vi "Teleop v1a.vi"(10 "Match Info":T1={"Autonomous Elapsed Seconds"=0.0, "TeleOp Elapsed Seconds"=0.0, "Disabled Elapsed Seconds"=0.0, "Visited Autonomous"=FALSE, "Visited TeleOp"=FALSE, "Visited Disabled"=FALSE, "Autonomous Settings"={"Autonomous Style"=enum."Independent", "VI Refnum"=refnum}}, 11 "Call Context":T2) -> ()   [LabVIEW 2019]
doc: "This VI is called for each TeleOp packet received from the DS where the robot is not disabled. It is often used to read from the joysticks and update I/O or to update setpoints for timed control loops. It should complete and return within 20 milliseconds or it may miss DS packets."
uses:
  <vilib>/Rock Robotics/WPI/DriverStation/WPI_DriverStationDerivedRobotMode.ctl
  <vilib>/Rock Robotics/WPI/DriverStation/WPI_DriverStationMatch Info.ctl
  <vilib>/Rock Robotics/WPI/Relay/WPI_RelayValue.ctl
  <vilib>/Rock Robotics/WPI/Utilities/WPI_GetSetVariantRefNum.vi
  <vilib>/Rock Robotics/Network Tables/NT Write Boolean Array.vi
  <vilib>/Rock Robotics/Network Tables/NT Write Numeric Array.vi
  <vilib>/Rock Robotics/Network Tables/NT Read Boolean.vi
  <vilib>/Rock Robotics/Network Tables/NT Read Number.vi
panel:
  out "Sample Slider 0":dbl(slide) scale=0.0..5.0
  out "Sample Boolean 1":bool
  out "Sample Boolean 0":bool
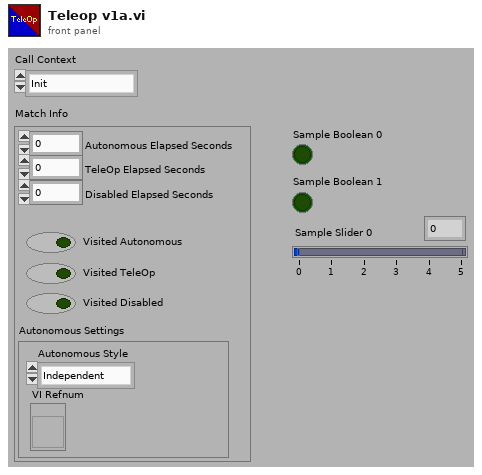
[diagram p1: front panel]
types:
  T1 = typedef "WPI_DriverStationMatch Info.ctl" = cluster{"Autonomous Elapsed Seconds":dbl, "TeleOp Elapsed Seconds":dbl, "Disabled Elapsed Seconds":dbl, "Visited Autonomous":bool, "Visited TeleOp":bool, "Visited Disabled":bool, "Autonomous Settings":cluster{"Autonomous Style":enum16{"Iterative", "Independent"}, "VI Refnum":refnum<vi>}}
  T2 = typedef "WPI_DriverStationDerivedRobotMode.ctl" = enum16{"Init", "Execute", "Stop"}
  T3 = typedef "WPI_RobotDriveDevRef.ctl" = cluster{"DevStatus":errorcluster, "Motors[]":T4[], "Square Inputs":bool, "Max Output":dbl}
  T4 = typedef "WPI_MotorControlDeviceRef.ctl" = cluster{"DeviceStatus":errorcluster, "Type":T5, "PWM":cluster{"PWM Channel":T6, "DeadBand":T7}, "CAN":cluster{"Device Number":u8, "SetOutput VI Ref":variant, "GetOutput VI Ref":variant, "Enable VI Ref":variant, "Disable VI Ref":variant, "Data":variant}, "Invert":bool, "DIO PWM":cluster{"PWM \"Enable\" Channel":T6, "DIOChannel":T8, "PWM Rate":dbl}}
  T5 = typedef "WPI_MotorControlType.ctl" = enum16{"PWM", "CAN", "DIO PWM"}
  T6 = typedef "FPGA_DIOPWMChannel.ctl" = enum8{"PWM 0", "PWM 1", "PWM 2", "PWM 3", "PWM 4", "PWM 5", "PWM 6", "PWM 7", "PWM 8", "PWM 9", "PWM MXP 0", "PWM MXP 1", "PWM MXP 2", "PWM MXP 3", "PWM MXP 4", "PWM MXP 5", "PWM MXP 6", "PWM MXP 7", "PWM MXP 8", "PWM MXP 9", "Invalid"}
  T7 = typedef "WPI_PWMDeadband.ctl" = cluster{"Name":string, "maxPositivePwm":i32, "minPositivePwm":i32, "centerPwm":i32, "maxNegativePwm":i32, "minNegativePwm":i32, "angularRange":u16}
  T8 = typedef "FPGA_DIOChannel.ctl" = enum8{"DIO 0", "DIO 1", "DIO 2", "DIO 3", "DIO 4", "DIO 5", "DIO 6", "DIO 7", "DIO 8", "DIO 9", "DIO MXP 0", "DIO MXP 1", "DIO MXP 2", "DIO MXP 3", "DIO MXP 4", "DIO MXP 5", "DIO MXP 6", "DIO MXP 7", "DIO MXP 8", "DIO MXP 9", "DIO MXP 10", "DIO MXP 11", "DIO MXP 12", "DIO MXP 13", "DIO MXP 14", "DIO MXP 15", "SPI Port CS1", "SPI Port CS2", "SPI Port CS3", "SPI Port MISO", "SPI Port MOSI", "Invalid"}
  T9 = typedef "WPI_JoystickDevRef.ctl" = cluster{"Device":T10}
  T10 = typedef "WPI_JoystickDeviceEnum.ctl" = enum16{"USB 0", "USB 1", "USB 2", "USB 3", "USB 4", "USB 5"}
  T11 = typedef "WPI_DigitalInputDevRef.ctl" = cluster{"DevStatus":errorcluster, "DIO Channel":T8}
  T12 = typedef "WPI_RelayValue.ctl" = enum16{"Off", "On", "Forward", "Reverse"}
  T13 = typedef "WPI_RelayDevRef.ctl" = cluster{"DevStatus":errorcluster, "Relay Channel":T14, "Relay Direction":T15}
  T14 = typedef "FPGA_DIORelayChannel.ctl" = enum8{"Relay 0", "Relay 1", "Relay 2", "Relay 3", "Invalid"}
  T15 = typedef "WPI_RelayDirection.ctl" = enum16{"Both directions", "Forward only", "Reverse only"}
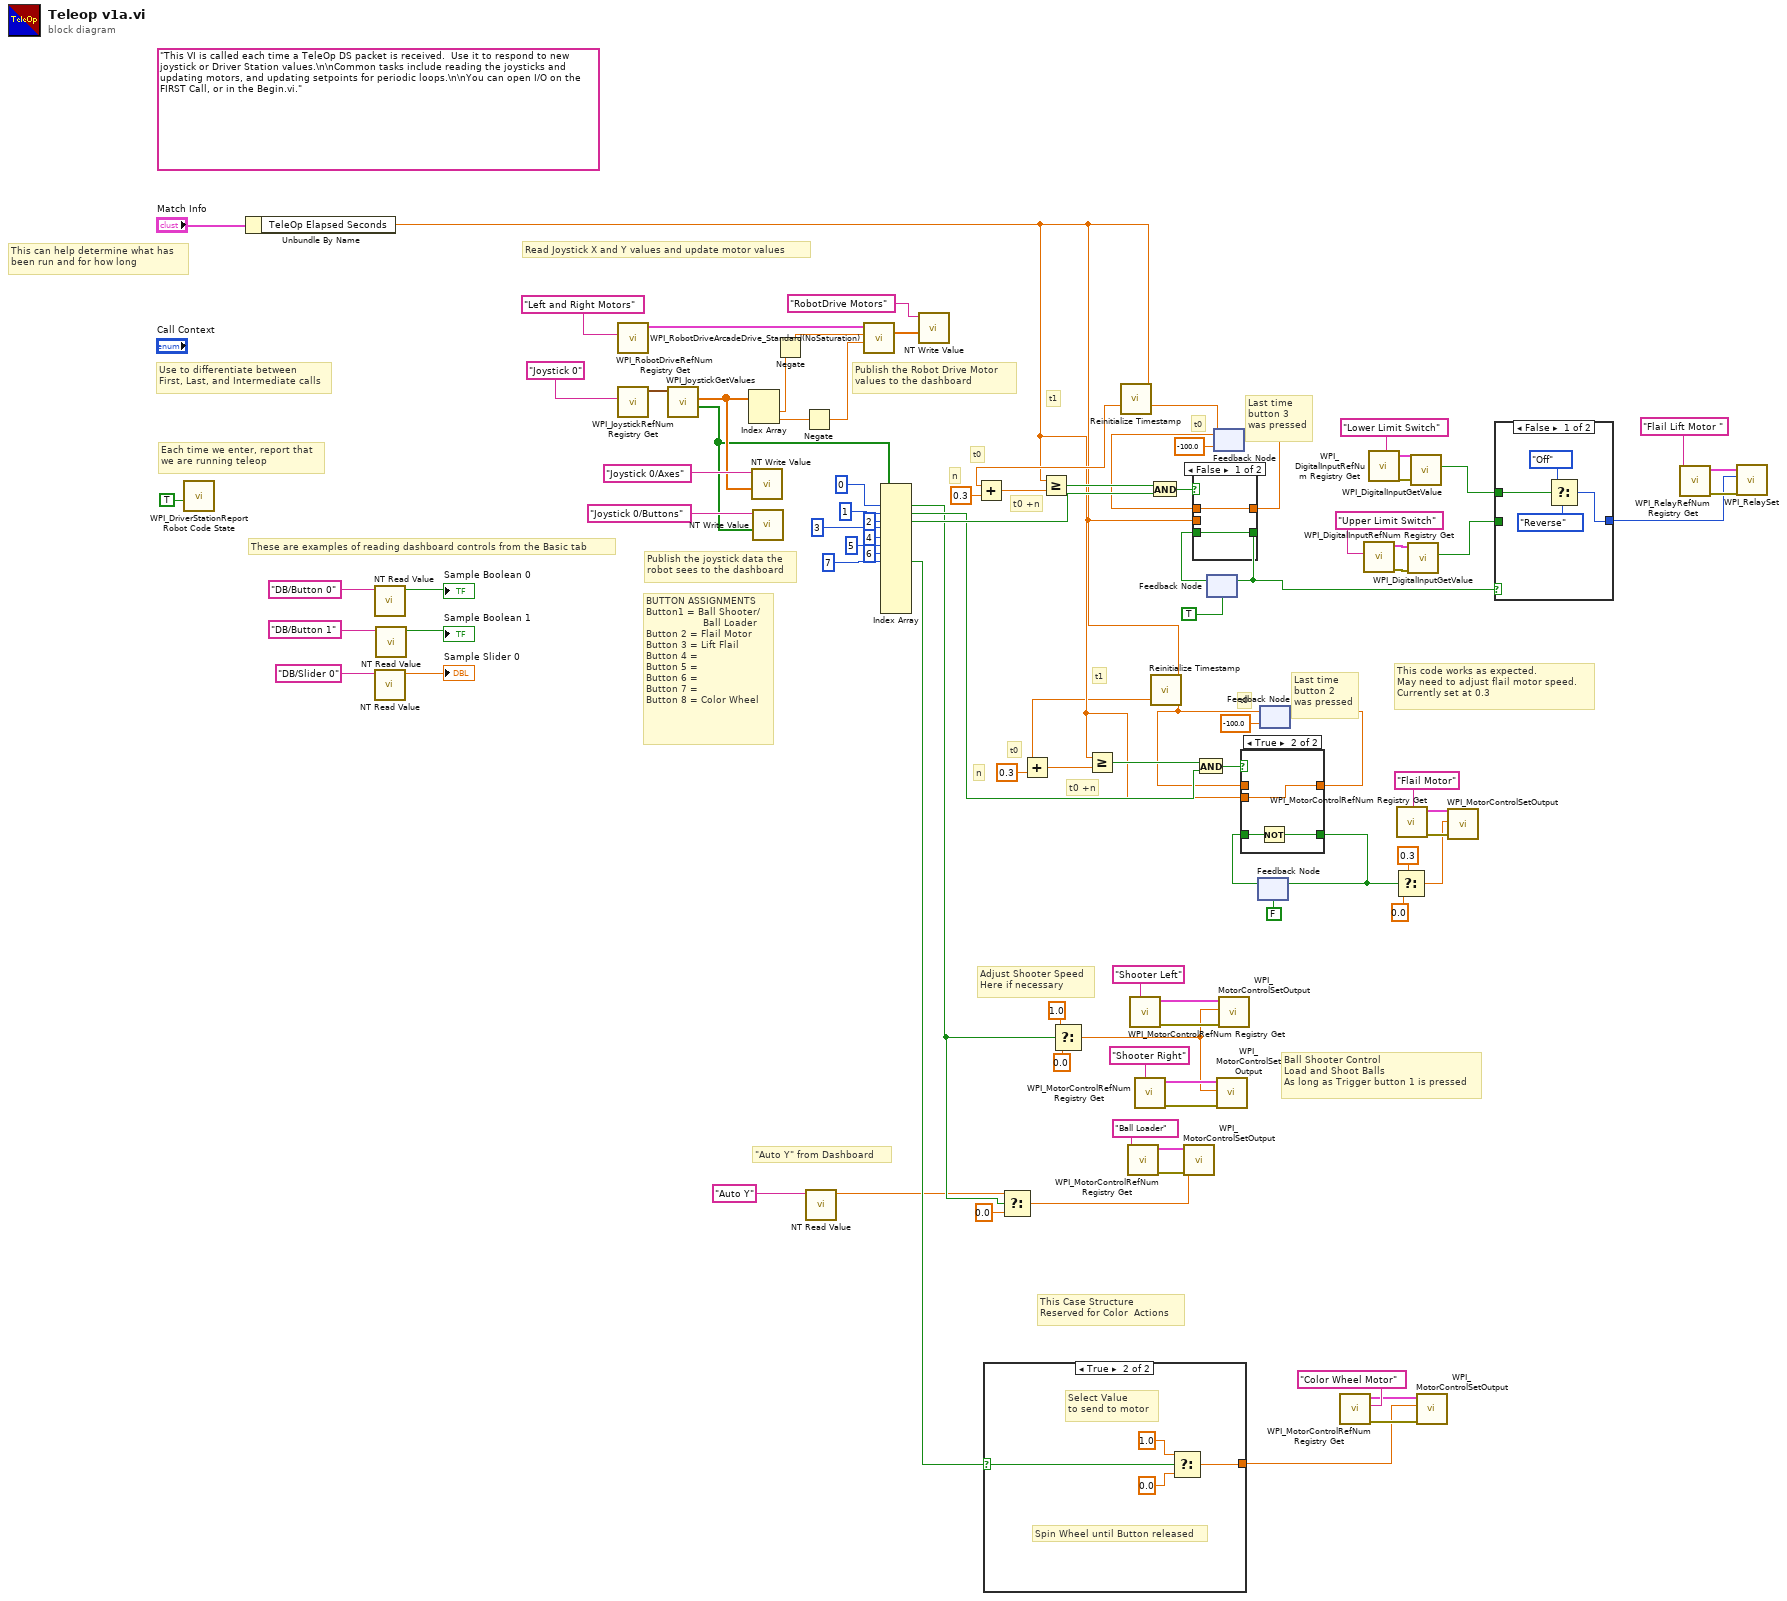
[diagram p0: block diagram]
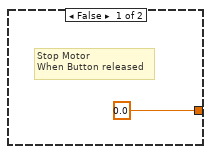
[diagram p2: hidden frame]
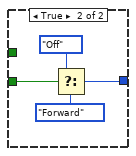
[diagram p4: hidden frame]
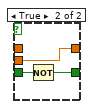
[diagram p5: hidden frame]
diagram:
  (unwired) "This VI is called each time a TeleOp DS packet is received.  Use it to respond to new joystick or Driver Station values.\n\nCommon tasks include reading the joysticks and updating motors, and updating setpoints for periodic loops.\n\nYou can open I/O on the FIRST Call, or in the Begin.vi."
  # "\"Auto Y\" from Dashboard"
  # "This Case Structure\nReserved for Color  Actions"
  # "Adjust Shooter Speed\nHere if necessary"
  # "Ball Shooter Control\nLoad and Shoot Balls \nAs long as Trigger button 1 is pressed"
  # "BUTTON ASSIGNMENTS\nButton1 = Ball Shooter/\n                   Ball Loader\nButton 2 = Flail Motor\nButton 3 = Lift Flail\nButton 4 =\nButton 5 = \nButton 6 =\nButton 7 =\nButton 8 = Color Wheel"
  # "This code works as expected.\nMay need to adjust flail motor speed.\nCurrently set at 0.3"
  # "n"
  # "t0"
  # "t0 +n"
  # "t0"
  # "t1"
  # "Last time \nbutton 2\nwas pressed"
  # "n"
  # "t0"
  # "t0 +n"
  # "t0"
  # "t1"
  # "Last time \nbutton 3\nwas pressed"
  # "These are examples of reading dashboard controls from the Basic tab"
  # "Publish the Robot Drive Motor\nvalues to the dashboard"
  # "Publish the joystick data the\nrobot sees to the dashboard"
  # "Each time we enter, report that\nwe are running teleop"
  # "Use to differentiate between\nFirst, Last, and Intermediate calls"
  # "This can help determine what has\nbeen run and for how long"
  # "Read Joystick X and Y values and update motor values"
  n1 = call <vilib>:"WPI_DriverStationReport Robot Code State.vi"("TeleOp"=TRUE ("Autonomous")) -> ()  [unwired: 10 in, 1 out]
  n2 = Unbundle By Name("Match Info") -> ("TeleOp Elapsed Seconds"=w6:dbl)
  n3 = call-poly <vilib>:"NT Read Value.vi"("Name"="DB/Button 0" ("refnum name")) -> ("Boolean"=→"Sample Boolean 0":bool)  [unwired: 9 in, 1 out]
  n4 = call-poly <vilib>:"NT Read Value.vi"("Name"="DB/Slider 0" ("refnum name")) -> ("Numeric"=→"Sample Slider 0":dbl)  [unwired: 9 in, 1 out]
  n5 = call-poly <vilib>:"NT Read Value.vi"("Name"="DB/Button 1" ("refnum name")) -> ("Boolean"=→"Sample Boolean 1":bool)  [unwired: 9 in, 1 out]
  n6 = call <vilib>:"WPI_RobotDriveRefNum Registry Get.vi"("refnum name"="Left and Right Motors") -> ("RobotDriveDevRef"=w93:T3)  [unwired: 1 in, 9 out]
  n7 = call <vilib>:"WPI_JoystickRefNum Registry Get.vi"("refnum name"="Joystick 0") -> ("JoystickDevRef"=w91:T9)  [unwired: 1 in, 9 out]
  n8 = call <vilib>:"WPI_JoystickGetValues.vi"("JoystickDevRef"=w91) -> ("Buttons"=w78:bool[], "Axes"=w87:dbl[])  [unwired: 6 in, 3 out]
  n9 = Index Array(array=w87) -> (element #1=w76:dbl, element #2=w75:dbl)  [unwired: 2 in]
  n10 = call-poly <vilib>:"NT Write Value.vi"("Numeric Array"=w87, "Name"="Joystick 0/Axes") -> ()  [unwired: 9 in, 1 out]
  n11 = call-poly <vilib>:"NT Write Value.vi"("Boolean Array"=w78, "Name"="Joystick 0/Buttons") -> ()  [unwired: 9 in, 1 out]
  n12 = Negate(x=w76) -> (-x=w2:dbl)
  n13 = Negate(x=w75) -> (-x=w3:dbl)
  n14 = call-poly <vilib>:"NT Read Value.vi"("Name"="Auto Y") -> ("Numeric"=w1:dbl)  [unwired: 9 in, 1 out]
  n15 = call <vilib>:"WPI_RobotDriveArcadeDrive_Standard(NoSaturation).vi"("Y axis value"=w3, "X axis value"=w2, "RobotDriveDevRef"=w93) -> ("Motor Values"=w80:dbl[])  [unwired: 1 in, 7 out]
  n16 = Index Array(array=w78, index #1=0 ("index"), index #2=1 ("index"), index #3=2 ("index"), index #4=3 ("index"), index #5=4 ("index"), index #6=5 ("index"), index #7=6 ("index"), index #8=7 ("index")) -> (element #1=w23:bool, element #2=w35:bool, element #3=w67:bool, element #8=w12:bool)  [unwired: 6 in, 10 out]
  n17 = call-poly <vilib>:"NT Write Value.vi"("Numeric Array"=w80, "Name"="RobotDrive Motors") -> ()  [unwired: 9 in, 1 out]
  n18 = case shown="True" w12 {
    selector: w12 -> [_ w100]
    tunnel: [0.0 ("f") w97] -> w18
    frame False {
      # "Stop Motor\nWhen Button released"
    }
    frame True {
      # "Spin Wheel until Button released"
      # "Select Value \nto send to motor"
      n19 = Select(t=1.0, s=w100, f=0.0) -> (s? t:f=w97:dbl)
    }
  }
  n20 = Select(t=w1, s=w23, f=0.0) -> (s? t:f=w9:dbl)
  n21 = Select(t=1.0, s=w23, f=0.0) -> (s? t:f=w28:dbl)
  n22 = call <vilib>:"WPI_MotorControlRefNum Registry Get.vi"("refnum name"="Ball Loader") -> ("error out"=w25:errorcluster, "MotorControlDevRef"=w24:T4)  [unwired: 9 in]
  n23 = call <vilib>:"WPI_MotorControlRefNum Registry Get.vi"("refnum name"="Shooter Left") -> ("error out"=w34:errorcluster, "MotorControlDevRef"=w33:T4)  [unwired: 9 in]
  n24 = call <vilib>:"WPI_MotorControlRefNum Registry Get.vi"("refnum name"="Shooter Right") -> ("error out"=w31:errorcluster, "MotorControlDevRef"=w30:T4)  [unwired: 9 in]
  n25 = call <vilib>:"WPI_MotorControlSetOutput.vi"("error in (no error)"=w25, "Output"=w9, "MotorControlDevRef"=w24) -> ()  [unwired: 6 in, 3 out]
  n26 = feedback #1(TRUE) -> (w73:bool)
  n27 = feedback #2(-100.0 ("TeleOp Elapsed Seconds")) -> (w7:dbl)
  n28 = call "Reinitialize Timestamp.vi"("t0 Input"=w7, "t1 Input"=w6) -> ("t0 Output"=w8:dbl)  [unwired: 9 in]
  n29 = Add(x=w8, y=0.3) -> (x+y=w65:dbl)
  n30 = Greater Or Equal?(x=w6, y=w65) -> (x >= y?=w62:bool)
  n31 = And(x=w62, y=w67) -> (x .and. y?=w66:bool)
  n32 = case shown="False" w66 {
    tunnel: [w102 w105] -> w52
    tunnel: w73 -> [w102 w104]
    tunnel: w7 -> [w101 _]
    tunnel: [w101 w103] -> w68
    tunnel: w6 -> [_ w103]
    frame False {
    }
    frame True {
      n33 = Not(x=w104) -> (.not. x?=w105:bool)
    }
  }
  n34 = feedback-in #1(w52) -> ()
  n35 = feedback-in #2(w68) -> ()
  n36 = call <vilib>:"WPI_MotorControlSetOutput.vi"("error in (no error)"=w31, "Output"=w28, "MotorControlDevRef"=w30) -> ()  [unwired: 6 in, 3 out]
  n37 = call <vilib>:"WPI_MotorControlSetOutput.vi"("error in (no error)"=w34, "Output"=w28, "MotorControlDevRef"=w33) -> ()  [unwired: 6 in, 3 out]
  n38 = feedback #3(FALSE) -> (w48:bool)
  n39 = feedback #4(-100.0 ("TeleOp Elapsed Seconds")) -> (w4:dbl)
  n40 = call "Reinitialize Timestamp.vi"("t0 Input"=w4, "t1 Input"=w6) -> ("t0 Output"=w5:dbl)  [unwired: 9 in]
  n41 = Add(x=w5, y=0.3) -> (x+y=w45:dbl)
  n42 = Greater Or Equal?(x=w6, y=w45) -> (x >= y?=w42:bool)
  n43 = And(x=w42, y=w35) -> (x .and. y?=w46:bool)
  n44 = case shown="True" w46 {
    tunnel: [w107 w110] -> w40
    tunnel: w48 -> [w107 w109]
    tunnel: w4 -> [w106 _]
    tunnel: [w106 w108] -> w47
    tunnel: w6 -> [_ w108]
    frame False {
    }
    frame True {
      n45 = Not(x=w109) -> (.not. x?=w110:bool)
    }
  }
  n46 = feedback-in #3(w40) -> ()
  n47 = feedback-in #4(w47) -> ()
  n48 = call <vilib>:"WPI_MotorControlRefNum Registry Get.vi"("refnum name"="Color Wheel Motor") -> ("error out"=w20:errorcluster, "MotorControlDevRef"=w19:T4)  [unwired: 9 in]
  n49 = call <vilib>:"WPI_DigitalInputRefNum Registry Get.vi"("refnum name"="Upper Limit Switch") -> ("error out"=w56:errorcluster, "DigitalInputDevRef"=w55:T11)  [unwired: 9 in]
  n50 = call <vilib>:"WPI_DigitalInputRefNum Registry Get.vi"("refnum name"="Lower Limit Switch") -> ("error out"=w60:errorcluster, "DigitalInputDevRef"=w59:T11)  [unwired: 9 in]
  n51 = Select(t=0.3, s=w40, f=0.0) -> (s? t:f=w37:dbl)
  n52 = call <vilib>:"WPI_MotorControlRefNum Registry Get.vi"("refnum name"="Flail Motor") -> ("error out"=w51:errorcluster, "MotorControlDevRef"=w50:T4)  [unwired: 9 in]
  n53 = call <vilib>:"WPI_DigitalInputGetValue.vi"("error in (no error)"=w56, "DigitalInputDevRef"=w55) -> ("Value"=w54:bool)  [unwired: 7 in, 2 out]
  n54 = call <vilib>:"WPI_DigitalInputGetValue.vi"("error in (no error)"=w60, "DigitalInputDevRef"=w59) -> ("Value"=w57:bool)  [unwired: 7 in, 2 out]
  n55 = call <vilib>:"WPI_MotorControlSetOutput.vi"("error in (no error)"=w20, "Output"=w18, "MotorControlDevRef"=w19) -> ()  [unwired: 6 in, 3 out]
  n56 = call <vilib>:"WPI_MotorControlSetOutput.vi"("error in (no error)"=w51, "Output"=w37, "MotorControlDevRef"=w50) -> ()  [unwired: 6 in, 3 out]
  n57 = case shown="False" w52 {
    tunnel: [w111 w116] -> w69
    tunnel: w57 -> [w112 _]
    tunnel: w54 -> [_ w115]
    frame False {
      n58 = Select(t=WPI_RelayValue."Off" ("RelayValue"), s=w112, f=WPI_RelayValue."Reverse" ("RelayValue")) -> (s? t:f=w111:T12)
    }
    frame True {
      n59 = Select(t=WPI_RelayValue."Off" ("RelayValue"), s=w115, f=WPI_RelayValue."Forward" ("RelayValue")) -> (s? t:f=w116:T12)
    }
  }
  n60 = call <vilib>:"WPI_RelayRefNum Registry Get.vi"("refnum name"="Flail Lift Motor ") -> ("error out"=w72:errorcluster, "RelayDevRef"=w71:T13)  [unwired: 9 in]
  n61 = call <vilib>:"WPI_RelaySet.vi"("error in (no error)"=w72, "RelayValue"=w69, "RelayDevRef"=w71) -> ()  [unwired: 7 in, 2 out]
